vi "Comm Constants.vi"() -> ()   [LabVIEW 2020, in "NI VeriStand Addon Network Comm Shared.lvlib"]
uses:
  NI VeriStand Addon Network Comm Shared.lvlib
panel:
  in  "ResponseQKey":string="RESPONSEQ"
  in  "ResponseSufix":string="_RESPONSE"
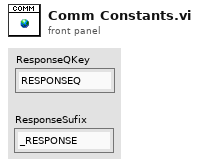
[diagram p1: front panel]
diagram:
